vi "vision communication serial port.vi"(8 "Invert Polarity?":bool, 11 "baud rate (9600)":u32=9600) -> ()   [LabVIEW 2010]
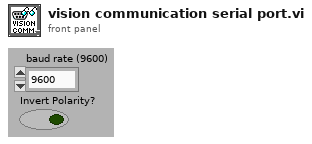
[diagram p1: front panel]
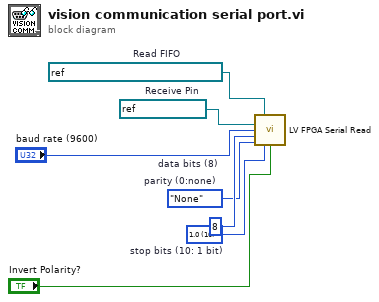
[diagram p0: block diagram]
diagram:
  w2 = u16 10 items=["1.0"=10, "1.5"=15, "2.0"=20]  # stop bits (10: 1 bit)
  w3 = enum16{"None", "Odd", "Even", "Mark", "Space"}."None"  # parity (0:none)
  w4 = 8  # data bits (8)
  w6 = refnum<k21> "Port4/DIO3"  # Receive Pin
  w7 = refnum<k21> "vision communication FIFO"  # Read FIFO
  n1 = call "LV FPGA Serial Read.vi"("Read FIFO"=w7, "Receive"=w6, "baud rate (9600)"="baud rate (9600)", "data bits (8)"=w4, "parity (0:none)"=w3, "stop bits (10: 1 bit)"=w2, "Invert Polarity?"="Invert Polarity?") -> ()  [unwired: 9 in]
